vi "simulationTest.vi"() -> ()   [LabVIEW 2021]
panel:
  out "Array 2":dbl[](array[numeric])
  in  "Array":dbl[](array[numeric])
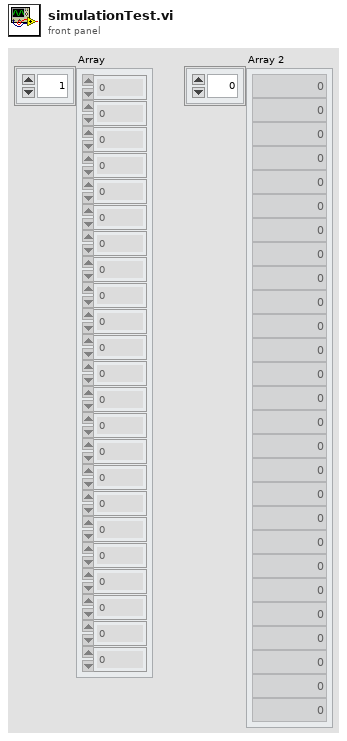
[diagram p1: front panel]
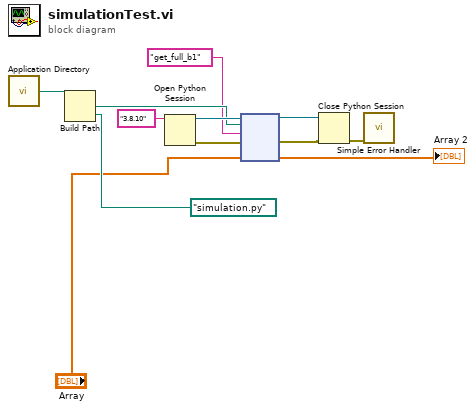
[diagram p0: block diagram]
diagram:
  n1 = call <vilib>:"Application Directory.vi"() -> ("Application Directory"=w7:path)
  n2 = Build Path(base path=w7, name or relative path=path "simulation.py") -> (appended path=w5:path)
  n3 = Open Python Session(python version="3.8.10" ("Python version")) -> (session out=w12:refnum<k35>, error out=w11:errorcluster)  [unwired: 2 in]
  n4 = node(w12, w5, "get_full_b1" ("function name"), w11, "Array") -> (w9:refnum<k35>, w10:errorcluster, →"Array 2":dbl[])  [unwired: 2 in, 2 out]
  n5 = Close Python Session(session in=w9, error in=w10) -> (11:w3:errorcluster)
  n6 = call <vilib>:"Simple Error Handler.vi"("error in (no error)"=w3) -> ()  [unwired: 4 in, 5 out]
